vi "StartTestSuite_WithTestSuite_AddsTestSuite.vi"() -> (0 "error out":errorcluster)   [LabVIEW 2017, in "ResultTreeListener.Tests.lvlib"]
uses:
  ResultTreeListener.Tests.lvlib
  6b75ad31-72ea-41ab-b928-28c96779d91c.vi
  Support/FakeTestSuite/FakeTestSuite.lvclass
  C:/Users/de200256/Code/logmanoriginal/lvunit/TestSuite/TestSuite.lvclass
  Constraint/IsEqual/Create.vi
  ResultTreeListener/ResultTreeListener.lvclass
  Constraint/IsEqual/IsEqual.lvclass
  ResultTree/ResultTree.lvclass
panel:
  in  "Tree":string(tree)
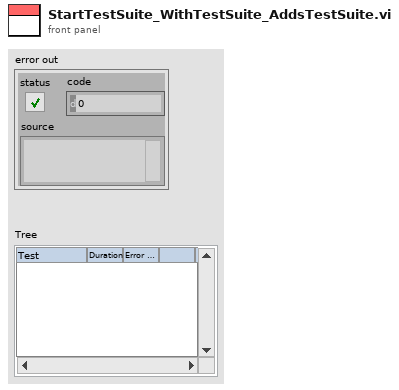
[diagram p1: front panel]
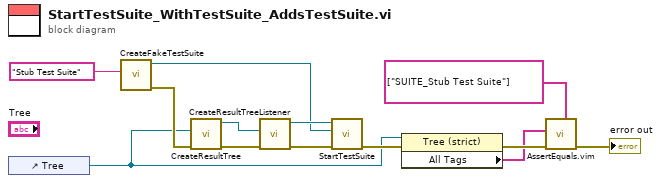
[diagram p0: block diagram]
diagram:
  n1 = control-ref of="Tree"() -> (w3:refnum<vi>)
  n2 = call "CreateFakeTestSuite.vi"("Name"="Stub Test Suite") -> ("error out"=w5:errorcluster, "FakeTestSuite out"=w7:refnum<class "FakeTestSuite.lvclass">)  [unwired: 9 in]
  n3 = call "CreateResultTree.vi"("error in (no error)"=w5, "Tree Refnum"=w3) -> ("error out"=w13:errorcluster, "ResultTree out"=w12:refnum<class "ResultTree.lvclass">)  [unwired: 8 in]
  n4 = call "CreateResultTreeListener.vi"("error in (no error)"=w13, "ResultTree"=w12) -> ("error out"=w11:errorcluster, "ResultTreeListener out"=w8:refnum<class "ResultTreeListener.lvclass">)  [unwired: 8 in]
  n5 = call-dynamic "StartTestSuite.vi"("error in (no error)"=w11, "TestSuite"=w7, "ResultTreeListener in"=w8) -> ("error out"=w9:errorcluster)  [unwired: 7 in, 1 out]
  n6 = property class="Tree (strict)"(reference=w3, error in=w9) -> (error out=w4:errorcluster, "All Tags"=w2:string[])  [unwired: 1 out]
  n7 = call "AssertEquals.vim"("Expected"=string[] ["SUITE_Stub Test Suite"] ("All Tags"), "error in (no error)"=w4, "Actual"=w2) -> ("error out"=→"error out":errorcluster)  [unwired: 8 in]
